vi "ZeroYaw.vi"(8 "error in (no error)":errorcluster, 11 "Nav6DevRef":T1) -> (0 "error out":errorcluster, 3 "Nav6DevRef Out":T1)   [LabVIEW 2014, in "Nav6.lvlib"]
doc: "Set the current Yaw to 0, used to reset the Yaw angle."
uses:
  Nav6.lvlib
  Nav6DevRef.ctl
  <vilib>/Rock Robotics/WPI/SerialPort/WPI_SerialPortRef.ctl
  Nav6Mode.ctl
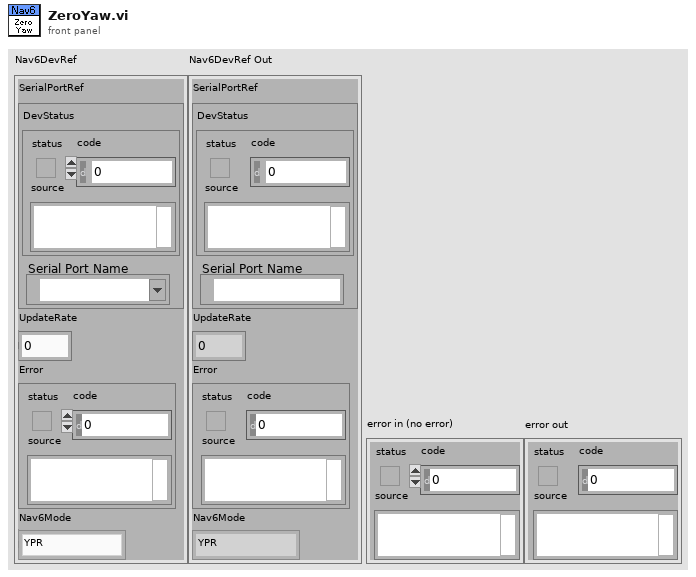
[diagram p1: front panel]
types:
  T1 = typedef "Nav6.lvlib/Nav6DevRef.ctl" = cluster{"SerialPortRef":T2, "UpdateRate":u8, "Error":errorcluster, "Nav6Mode":T3}
  T2 = typedef "WPI_SerialPortRef.ctl" = cluster{"DevStatus":errorcluster, "Serial Port Name":refnum<visa-resource-name>}
  T3 = typedef "Nav6.lvlib/Nav6Mode.ctl" = enum16{"YPR", "Gyro", "Quaternion"}
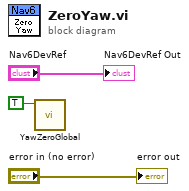
[diagram p0: block diagram]
diagram:
  n1 = call "YawZeroGlobal.vi"("Update"=TRUE) -> ()  [unwired: 10 in, 1 out]
  "Nav6DevRef Out" <- "Nav6DevRef"
  "error out" <- "error in (no error)"
